vi "PLC.Dial750, Get Config.vi"(7 "Config Folder":path=path "C:/MTE/Circle Test/Config", 8 "error in (no error)":errorcluster, 10 "VarNames In":T1={"SN"="g.SN", "Nest"="g.Nest", "Ready"="g.Ready", "Start"="g.Start", "Pass"="g.Pass", "Done"="g.Done", "Running"="GVL.gDone"}, 11 "Connection Info In":T2={"Net ID Target"="5.49.203.74.1.1", "Net ID Source"="192.168.1.18.1.1", "IP Address Target"="172.16.113.5", "Target Port"=851}) -> (0 "error out":errorcluster, 2 "VarNames":T1={"SN"="g.SN", "Nest"="g.Nest", "Ready"="g.Ready", "Start"="g.Start", "Pass"="g.Pass", "Done"="g.Done", "Running"="GVL.gDone"}, 3 "Connection Info":T2={"Net ID Target"="5.49.203.74.1.1", "Net ID Source"="192.168.1.18.1.1", "IP Address Target"="172.16.113.5", "Target Port"=851})   [LabVIEW 2018]
uses:
  Controls/PLC750.Connection Config.ctl
  Controls/PLC750.Variable Names.ctl
  <vilib>/Utility/config.llb/Read Key (String).vi
  <vilib>/Utility/config.llb/Read Key (U32).vi
  <vilib>/Utility/config.llb/NI_LVConfig.lvlib
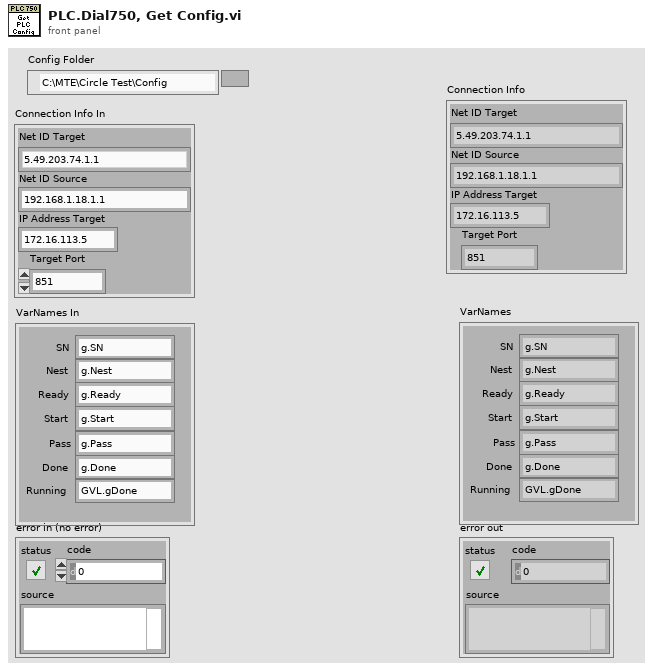
[diagram p1: front panel]
types:
  T1 = typedef "PLC750.Variable Names.ctl" = cluster{"SN":string, "Nest":string, "Ready":string, "Start":string, "Pass":string, "Done":string, "Running":string}
  T2 = typedef "PLC750.Connection Config.ctl" = cluster{"Net ID Target":string, "Net ID Source":string, "IP Address Target":string, "Target Port":u16}
  T3 = typedef "NI_LVConfig.lvlib/Config Data RefNum.ctl" = refnum<k1>
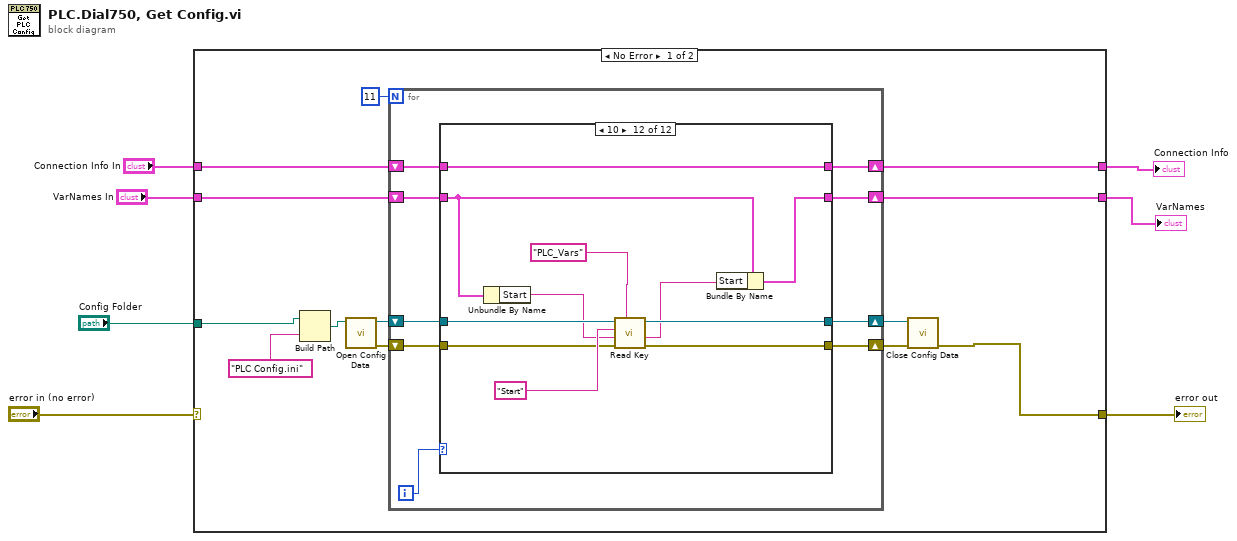
[diagram p0: block diagram]
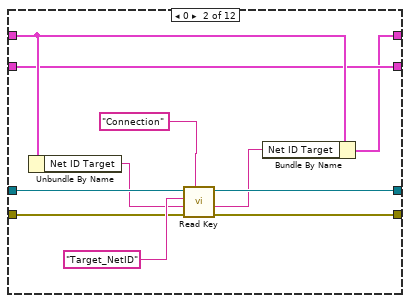
[diagram p3: hidden frame]
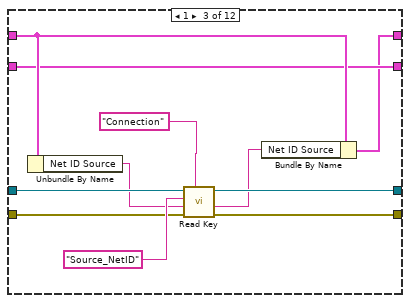
[diagram p4: hidden frame]
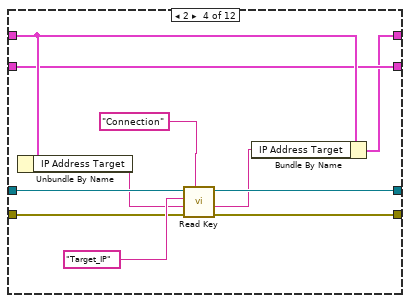
[diagram p5: hidden frame]
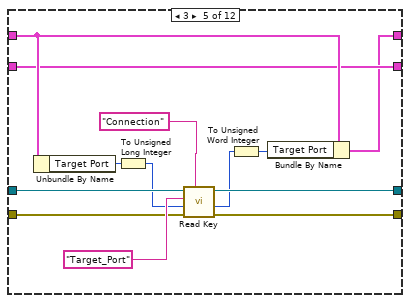
[diagram p6: hidden frame]
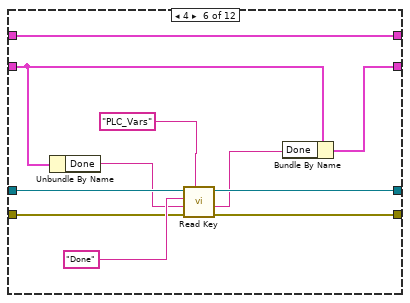
[diagram p7: hidden frame]
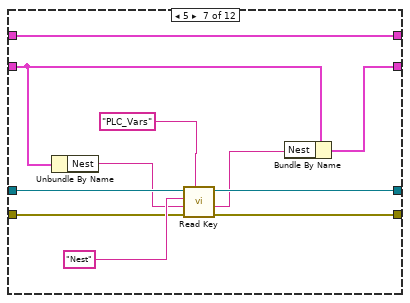
[diagram p8: hidden frame]
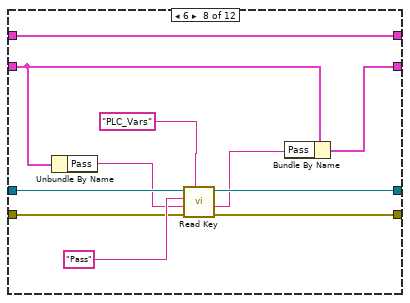
[diagram p9: hidden frame]
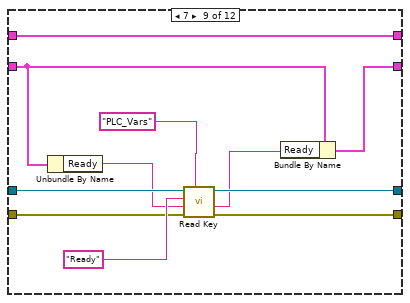
[diagram p10: hidden frame]
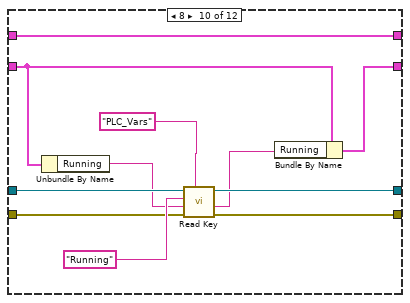
[diagram p11: hidden frame]
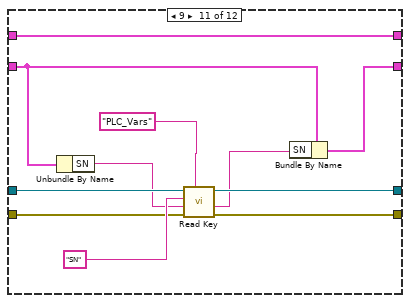
[diagram p12: hidden frame]
diagram:
  n1 = case shown="No Error" "error in (no error)" {
    selector: "error in (no error)" -> [_ w159]
    tunnel: [w11 w159] -> w6
    tunnel: "Connection Info In" -> [w16 w158]
    tunnel: "VarNames In" -> [w15 w157]
    tunnel: [w14 w158] -> w3
    tunnel: [w13 w157] -> w2
    tunnel: "Config Folder" -> [w9 _]
    frame No Error {
      n2 = Build Path(base path=w9, name or relative path="PLC Config.ini") -> (appended path=w10:path)
      n3 = call <vilib>:"Open Config Data.vi"("configuration file path"=w10) -> ("error out"=w20:errorcluster, "refnum"=w18:T3)  [unwired: 8 in, 1 out]
      n4 = for {
        N: 11 -> [_]
        shift-right: [w27] -> w19
        shift-left: w20 -> [w28]
        shift-right: [w25] -> w17
        shift-left: w18 -> [w26]
        shift-right: [w21] -> w14
        shift-left: w16 -> [w24]
        shift-right: [w22] -> w13
        shift-left: w15 -> [w23]
        i -> [w29]
        n5 = case shown="10" w29 {
          tunnel: w28 -> [w30 w42 w53 w64 w77 w88 w99 w110 w121 w132 w143 w154]
          tunnel: [w30 w41 w52 w63 w76 w87 w98 w109 w120 w131 w142 w153] -> w27
          tunnel: w26 -> [w31 w40 w51 w62 w75 w86 w97 w108 w119 w130 w141 w152]
          tunnel: [w31 w39 w50 w61 w74 w85 w96 w107 w118 w129 w140 w151] -> w25
          tunnel: w24 -> [w32 w37 w48 w59 w73 w84 w95 w106 w117 w128 w139 w150]
          tunnel: w23 -> [w33 w36 w47 w58 w72 w82 w93 w104 w115 w126 w137 w148]
          tunnel: [w33 w36 w47 w58 w72 w81 w92 w103 w114 w125 w136 w147] -> w22
          tunnel: [w32 w34 w45 w56 w71 w84 w95 w106 w117 w128 w139 w150] -> w21
          frame Default {
          }
          frame 0 {
            n6 = Unbundle By Name(w37) -> ("Net ID Target"=w38:string)
            n7 = call-poly <vilib>:"Read Key.vi"("section"="Connection", "error in (no error)"=w42, "default value"=w38, "key"="Target_NetID", "refnum"=w40) -> ("error out"=w41:errorcluster, "value"=w35:string, "refnum out"=w39:T3)  [unwired: 3 in, 1 out]
            n8 = Bundle By Name(cluster=w37, "Net ID Target"=w35) -> (w34:T2)
          }
          frame 1 {
            n9 = Unbundle By Name(w48) -> ("Net ID Source"=w49:string)
            n10 = call-poly <vilib>:"Read Key.vi"("section"="Connection", "error in (no error)"=w53, "default value"=w49, "key"="Source_NetID", "refnum"=w51) -> ("error out"=w52:errorcluster, "value"=w46:string, "refnum out"=w50:T3)  [unwired: 3 in, 1 out]
            n11 = Bundle By Name(cluster=w48, "Net ID Source"=w46) -> (w45:T2)
          }
          frame 2 {
            n12 = Unbundle By Name(w59) -> ("IP Address Target"=w60:string)
            n13 = call-poly <vilib>:"Read Key.vi"("section"="Connection", "error in (no error)"=w64, "default value"=w60, "key"="Target_IP", "refnum"=w62) -> ("error out"=w63:errorcluster, "value"=w57:string, "refnum out"=w61:T3)  [unwired: 3 in, 1 out]
            n14 = Bundle By Name(cluster=w59, "IP Address Target"=w57) -> (w56:T2)
          }
          frame 3 {
            n15 = Unbundle By Name(w73) -> ("Target Port"=w67:u16)
            n16 = To Unsigned Long Integer(number=w67) -> (unsigned 32bit integer=w68:u32)
            n17 = call-poly <vilib>:"Read Key.vi"("section"="Connection", "error in (no error)"=w77, "default value"=w68, "key"="Target_Port", "refnum"=w75) -> ("error out"=w76:errorcluster, "value"=w69:u32, "refnum out"=w74:T3)  [unwired: 3 in, 1 out]
            n18 = To Unsigned Word Integer(number=w69) -> (unsigned 16bit integer=w70:u16)
            n19 = Bundle By Name(cluster=w73, "Target Port"=w70) -> (w71:T2)
          }
          frame 4 {
            n20 = Unbundle By Name(w82) -> ("Done"=w83:string)
            n21 = call-poly <vilib>:"Read Key.vi"("section"="PLC_Vars", "error in (no error)"=w88, "default value"=w83, "key"="Done", "refnum"=w86) -> ("error out"=w87:errorcluster, "value"=w80:string, "refnum out"=w85:T3)  [unwired: 3 in, 1 out]
            n22 = Bundle By Name(cluster=w82, "Done"=w80) -> (w81:T1)
          }
          frame 5 {
            n23 = Unbundle By Name(w93) -> ("Nest"=w94:string)
            n24 = call-poly <vilib>:"Read Key.vi"("section"="PLC_Vars", "error in (no error)"=w99, "default value"=w94, "key"="Nest", "refnum"=w97) -> ("error out"=w98:errorcluster, "value"=w91:string, "refnum out"=w96:T3)  [unwired: 3 in, 1 out]
            n25 = Bundle By Name(cluster=w93, "Nest"=w91) -> (w92:T1)
          }
          frame 6 {
            n26 = Unbundle By Name(w104) -> ("Pass"=w105:string)
            n27 = call-poly <vilib>:"Read Key.vi"("section"="PLC_Vars", "error in (no error)"=w110, "default value"=w105, "key"="Pass", "refnum"=w108) -> ("error out"=w109:errorcluster, "value"=w102:string, "refnum out"=w107:T3)  [unwired: 3 in, 1 out]
            n28 = Bundle By Name(cluster=w104, "Pass"=w102) -> (w103:T1)
          }
          frame 7 {
            n29 = Unbundle By Name(w115) -> ("Ready"=w116:string)
            n30 = call-poly <vilib>:"Read Key.vi"("section"="PLC_Vars", "error in (no error)"=w121, "default value"=w116, "key"="Ready", "refnum"=w119) -> ("error out"=w120:errorcluster, "value"=w113:string, "refnum out"=w118:T3)  [unwired: 3 in, 1 out]
            n31 = Bundle By Name(cluster=w115, "Ready"=w113) -> (w114:T1)
          }
          frame 8 {
            n32 = Unbundle By Name(w126) -> ("Running"=w127:string)
            n33 = call-poly <vilib>:"Read Key.vi"("section"="PLC_Vars", "error in (no error)"=w132, "default value"=w127, "key"="Running", "refnum"=w130) -> ("error out"=w131:errorcluster, "value"=w124:string, "refnum out"=w129:T3)  [unwired: 3 in, 1 out]
            n34 = Bundle By Name(cluster=w126, "Running"=w124) -> (w125:T1)
          }
          frame 9 {
            n35 = Unbundle By Name(w137) -> ("SN"=w138:string)
            n36 = call-poly <vilib>:"Read Key.vi"("section"="PLC_Vars", "error in (no error)"=w143, "default value"=w138, "key"="SN", "refnum"=w141) -> ("error out"=w142:errorcluster, "value"=w135:string, "refnum out"=w140:T3)  [unwired: 3 in, 1 out]
            n37 = Bundle By Name(cluster=w137, "SN"=w135) -> (w136:T1)
          }
          frame 10 {
            n38 = Unbundle By Name(w148) -> ("Start"=w149:string)
            n39 = call-poly <vilib>:"Read Key.vi"("section"="PLC_Vars", "error in (no error)"=w154, "default value"=w149, "key"="Start", "refnum"=w152) -> ("error out"=w153:errorcluster, "value"=w146:string, "refnum out"=w151:T3)  [unwired: 3 in, 1 out]
            n40 = Bundle By Name(cluster=w148, "Start"=w146) -> (w147:T1)
          }
        }
      }
      n41 = call <vilib>:"Close Config Data.vi"("error in (no error)"=w19, "refnum"=w17) -> ("error out"=w11:errorcluster)  [unwired: 8 in, 1 out]
    }
    frame Error {
    }
  }
  "error out" <- w6
  "Connection Info" <- w3
  "VarNames" <- w2
